vi "GetNamedRendezvousPrefix.vi"() -> (2 "Named Semaphore Prefix":string)   [LabVIEW 2010]
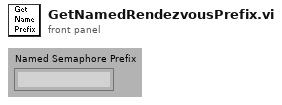
[diagram p1: front panel]
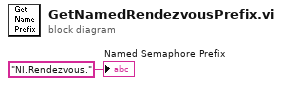
[diagram p0: block diagram]
diagram:
  "Named Semaphore Prefix" <- "NI.Rendezvous." ("Named Semaphore Prefix")
